vi "Latest Joystick State.vi"(8 "error in (no error)":errorcluster, 10 "Joystick State":cluster{"Buttons":T1[], "Axis":T2[]}, 11 "Driver in":refnum<class "Driver.lvclass">) -> (0 "error out":errorcluster, 3 "Driver out":refnum<class "Driver.lvclass">)   [LabVIEW 2014, in "Driver.lvlib" / "Driver.lvclass"]
uses:
  Driver.lvclass
  Joystick/Joystick Class/Button State.ctl
  Joystick/Joystick Class/Axis State.ctl
  Joystick/Joystick Class/Joystick.lvclass
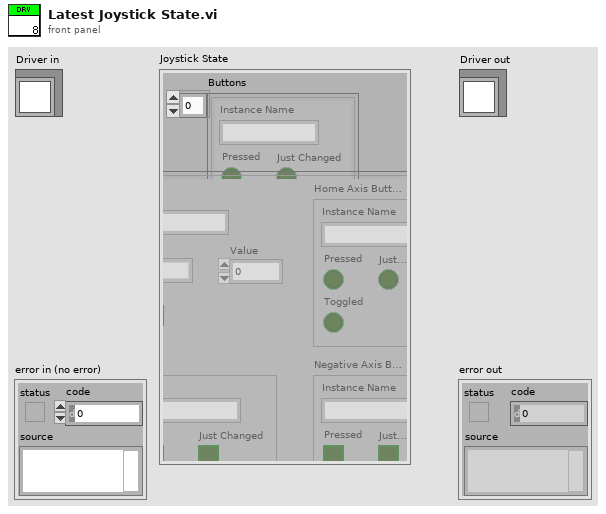
[diagram p1: front panel]
types:
  T1 = typedef "Joystick.lvlib/Joystick.lvclass/Button State.ctl" = cluster{"Pressed":bool, "Instance Name":string, "Toggled":bool, "Just Changed":bool}
  T2 = typedef "Joystick.lvlib/Joystick.lvclass/Axis State.ctl" = cluster{"Instance Name":string, "Deadband":dbl, "Value":dbl, "At Home":bool, "Postive Axis Button State":T1, "Negative Axis Button State":T1, "Home Axis Button State":T1}
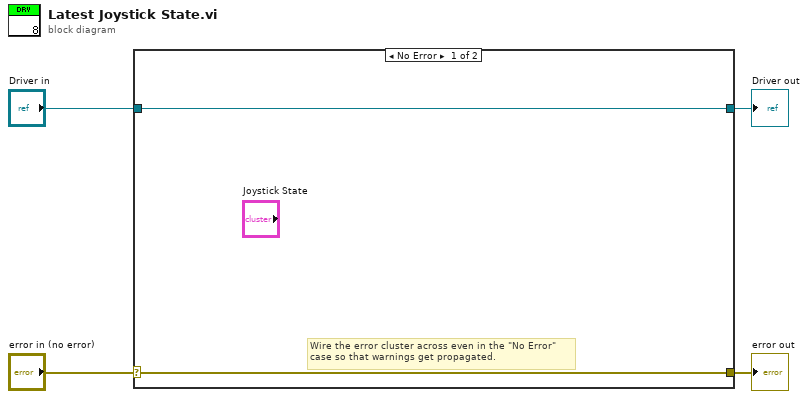
[diagram p0: block diagram]
diagram:
  n1 = case shown="No Error" "error in (no error)" {
    selector: "error in (no error)" -> [w5 w8]
    tunnel: [w5 w8] -> w3
    tunnel: [w6 w7] -> w1
    tunnel: "Driver in" -> [w6 w7]
    frame No Error {
      # "Wire the error cluster across even in the \"No Error\"\ncase so that warnings get propagated."
    }
    frame Error {
    }
  }
  "error out" <- w3
  "Driver out" <- w1
